vi "SLSC_Module_Session_Init.vi"(5 "Password":string, 6 "connect timeout (10 sec)":dbl=10.0, 7 "Username":string="admin", 8 "Error In":errorcluster, 10 "Slot #":u32=4, 11 "Chassis IP Address":string="192.168.0.14") -> (0 "Error Out":errorcluster, 1 "SLSC Chassis Name":string, 2 "SLSC Module Name":string, 3 "Module Session Out":string)   [LabVIEW 2015, in "SLSC-12201 DIO Engine.lvlib"]
uses:
  SLSC-12201 DIO Engine.lvlib
  <vilib>/nisyscfg/Close (System).vi
  <vilib>/SLSC/Initialize Session with Devices.vi
  <vilib>/SLSC/Initialize Session without Resources.vi
  <vilib>/SLSC/Close Session.vi
  <vilib>/SLSC/SLSC.lvlib
  <resource>/objmgr/slsc.rc
  <vilib>/nisyscfg/nisyscfg.lvlib
  <resource>/objmgr/nisysapi.rc
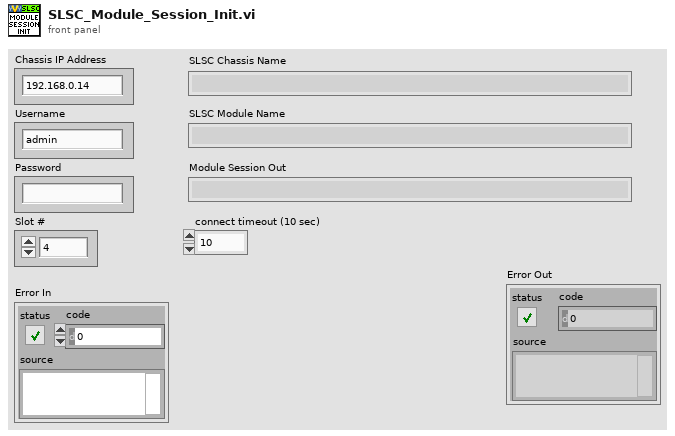
[diagram p1: front panel]
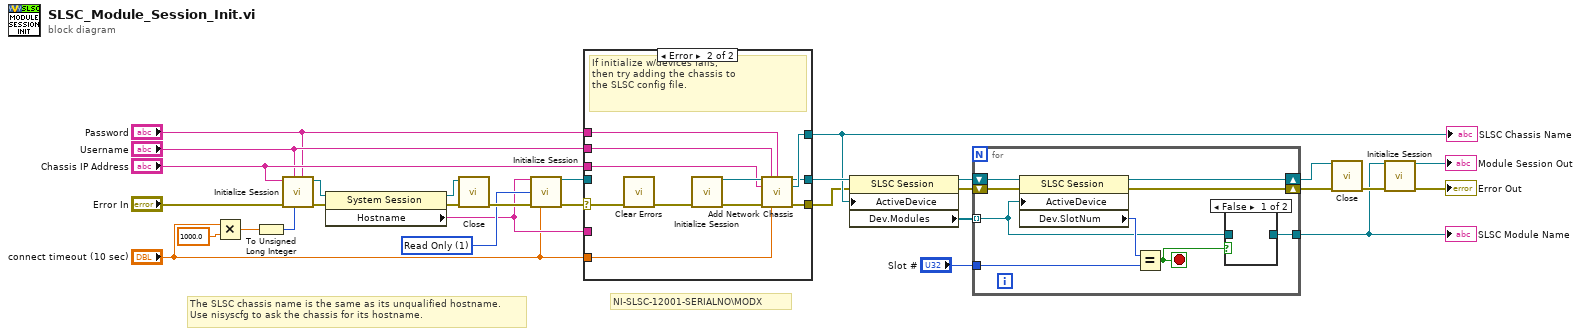
[diagram p0: block diagram]
diagram:
  w16 = 1 items=["None"=0, "Read Only"=1, "Read/Write"=3] ("reservation access (Read/Write)")
  # "NI-SLSC-12001-SERIALNO\\MODX"
  # "The SLSC chassis name is the same as its unqualified hostname.\nUse nisyscfg to ask the chassis for its hostname."
  n1 = Multiply(x="connect timeout (10 sec)", y=1000.0) -> (x*y=w11:dbl)
  n2 = To Unsigned Long Integer(number=w11) -> (unsigned 32bit integer=w10:u32)
  n3 = call <vilib>:"Initialize Session.vi"("Password"="Password", "Connect Timeout (4000 ms)"=w10, "User Name"="Username", "error in (no error)"="Error In", "Target (localhost)"="Chassis IP Address") -> ("error out"=w20:errorcluster, "Session out"=w21:refnum<k21>)  [unwired: 5 in]
  n4 = property class="System Session"(reference=w21, error in=w20) -> (reference out=w18:refnum<k21>, error out=w19:errorcluster, "Hostname"=w13:string)
  n5 = call-poly <vilib>:"Close.vi"("error in (no error)"=w19, "Session in"=w18) -> ("error out"=w17:errorcluster)  [unwired: 9 in]
  n6 = call-poly <vilib>:"Initialize Session.vi"("devices"=w13, "reservation access (Read/Write)"=w16, "error in (no error)"=w17, "connect timeout (60 sec)"="connect timeout (10 sec)") -> ("session out"=w14:refnum<k21>, "error out"=w15:errorcluster)  [unwired: 10 in]
  n7 = case shown="Error" w15 {
    selector: w15 -> [w33 w44]
    tunnel: [w33 w36] -> w3
    tunnel: [w32 w37] -> w5
    tunnel: w14 -> [w32 _]
    tunnel: "Chassis IP Address" -> [_ w42]
    tunnel: "Username" -> [_ w40]
    tunnel: "Password" -> [_ w39]
    tunnel: [w31 w38] -> w4
    tunnel: w13 -> [w31 _]
    tunnel: "connect timeout (10 sec)" -> [_ w34]
    frame No Error {
      # "If initialize w/devices succeeds,\nthen the SLSC driver already\nknows about this chassis via\nmDNS or the config file."
    }
    frame Error {
      # "If initialize w/devices fails,\nthen try adding the chassis to\nthe SLSC config file."
      n8 = call <vilib>:"Clear Errors.vi"("error in (no error)"=w44) -> ("error out"=w35:errorcluster)  [unwired: 5 in, 1 out]
      n9 = call-poly <vilib>:"Initialize Session.vi"("error in (no error)"=w35) -> ("session out"=w43:refnum<k21>, "error out"=w41:errorcluster)  [unwired: 13 in]
      n10 = call <vilib>:"Add Network Chassis.vi"("session in"=w43, "username"=w40, "password"=w39, "chassis IP address/hostname"=w42, "error in (no error)"=w41, "connect timeout (60 sec)"=w34) -> ("session out"=w37:refnum<k21>, "chassis out"=w38:refnum<k21>, "error out"=w36:errorcluster)  [unwired: 7 in]
    }
  }
  "SLSC Chassis Name" <- w4
  n11 = property class="SLSC Session"(reference=w5, error in=w3, "ActiveDevice"=w4) -> (reference out=w28:refnum<k21>, error out=w27:errorcluster, "Dev.Modules"=w30:refnum<k21>[])
  n12 = for {
    tunnel: w30 -> [w47] mode=indexing
    tunnel: "Slot #" -> [w53]
    tunnel: [w46] -> w24
    shift-right: [w49] -> w2
    shift-left: w27 -> [w50]
    shift-right: [w48] -> w26
    shift-left: w28 -> [w52]
    stop <- w45 stop-if-true
    n13 = property class="SLSC Session"(reference=w52, error in=w50, "ActiveDevice"=w47) -> (reference out=w48:refnum<k21>, error out=w49:errorcluster, "Dev.SlotNum"=w51:u32)
    n14 = Equal?(x=w51, y=w53) -> (x = y?=w45:bool)
    n15 = case shown="False" w45 {
      tunnel: w47 -> [_ w54]
      tunnel: [_ w54] -> w46
      frame False {
      }
      frame True {
      }
    }
  }
  "SLSC Module Name" <- w24
  n16 = call-poly <vilib>:"Close.vi"("session in"=w26, "error in (no error)"=w2) -> ("error out"=w25:errorcluster)  [unwired: 13 in]
  n17 = call-poly <vilib>:"Initialize Session.vi"("devices"=w24, "error in (no error)"=w25) -> ("session out"=→"Module Session Out":refnum<k21>, "error out"=→"Error Out":errorcluster)  [unwired: 12 in]
